vi "HandleObservation.vi"(8 "error in (no error)":errorcluster, 11 "S4ACS_GUI in":refnum<class "S4GUI.lvclass">) -> (0 "error out":errorcluster, 3 "S4ACS_GUI out":refnum<class "S4GUI.lvclass">)   [LabVIEW 2018, in "S4GUI.lvclass"]
uses:
  S4GUI.lvclass
  S4GUI.lvclass/S4GUI.ctl
  Acquisition/Acquisition.lvclass
  Trigger/Trigger.lvclass
  SyncBox/Sync Box.lvclass
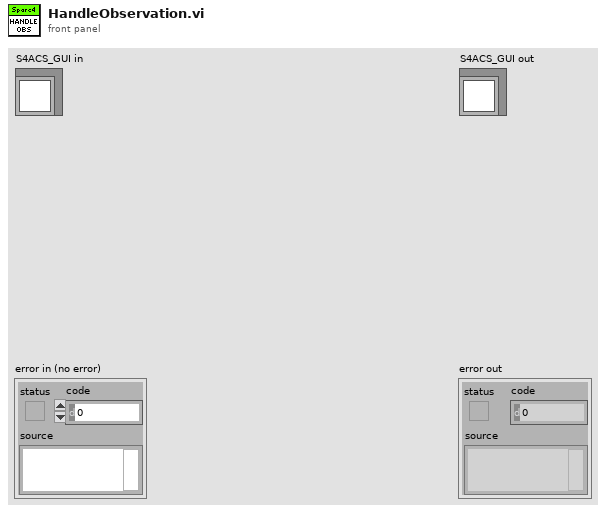
[diagram p1: front panel]
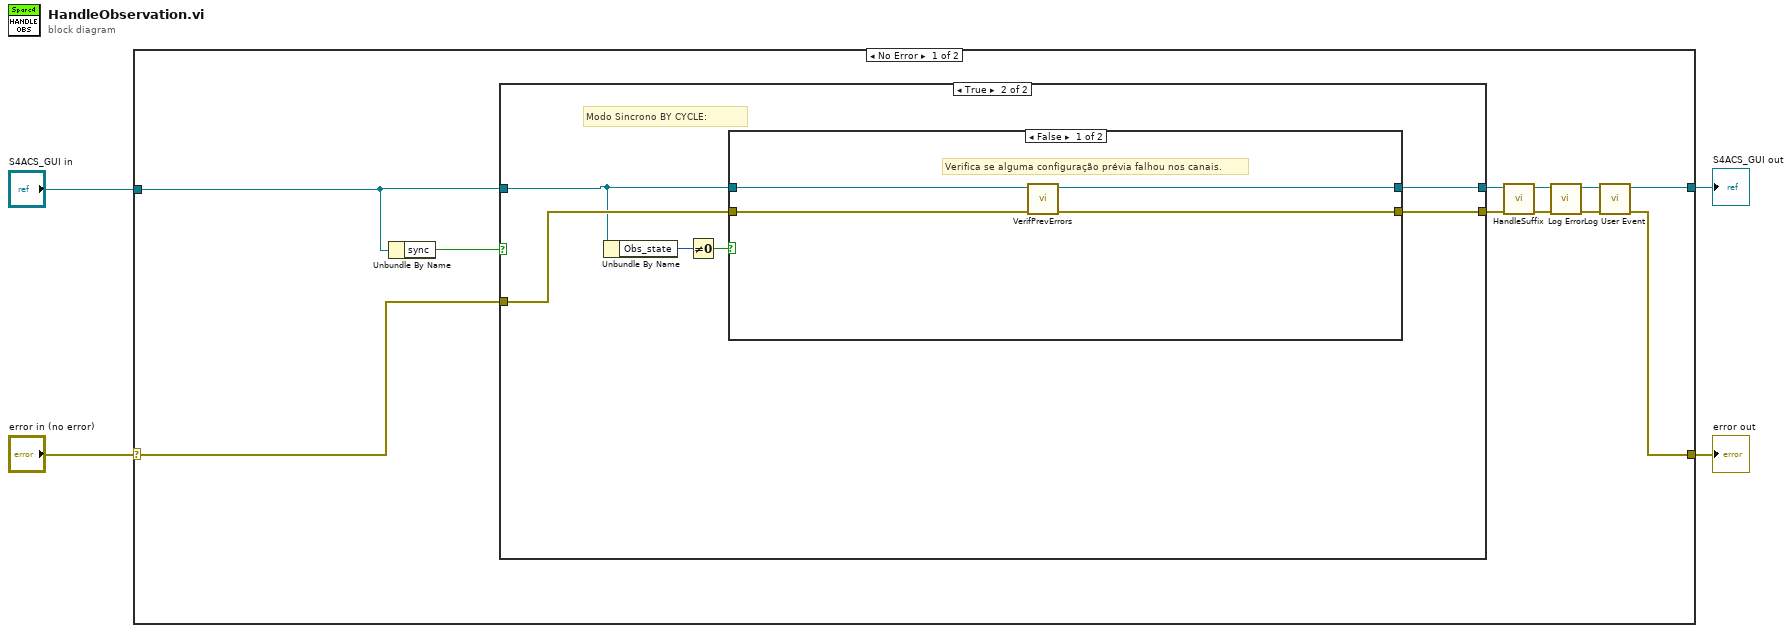
[diagram p0: block diagram]
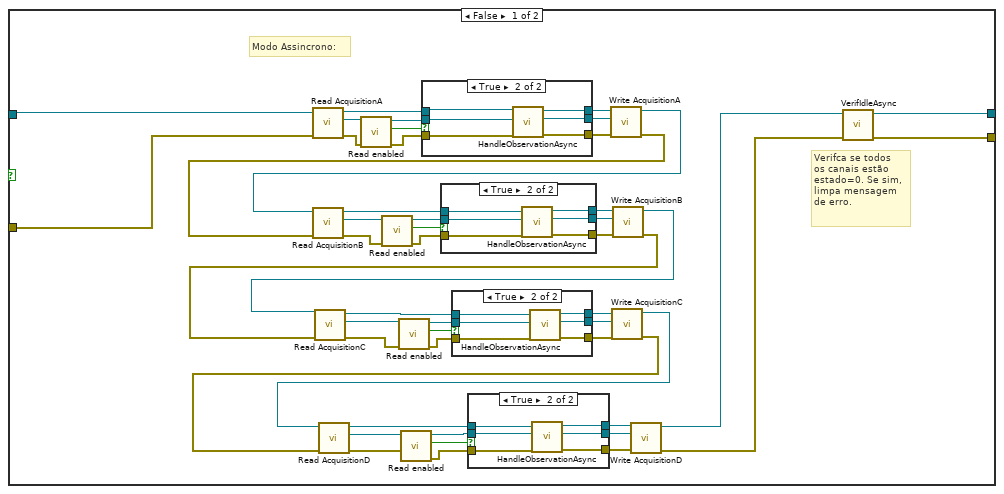
[diagram p2: hidden frame]
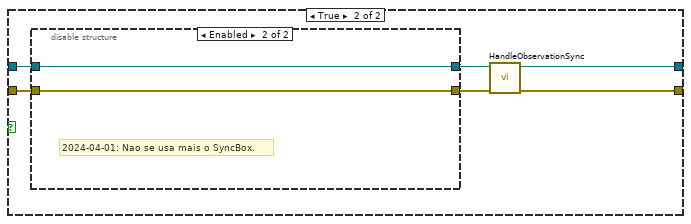
[diagram p7: hidden frame]
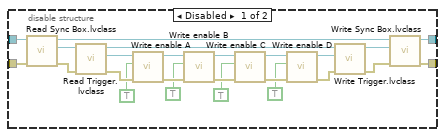
[diagram p8: hidden frame]
diagram:
  n1 = case shown="No Error" "error in (no error)" {
    selector: "error in (no error)" -> [w13 w143]
    tunnel: [w9 w143] -> w3
    tunnel: [w10 w142] -> w1
    tunnel: "S4ACS_GUI in" -> [w15 w142]
    frame No Error {
      n2 = Unbundle By Name(w15) -> ("sync"=w14:bool)
      n3 = case shown="True" w14 {
        tunnel: w15 -> [w27 w102]
        tunnel: [w17 w105] -> w8
        tunnel: w13 -> [w26 w103]
        tunnel: [w16 w104] -> w6
        frame False {
          # "Verifca se todos\nos canais estão \nestado=0. Se sim,\nlimpa mensagem \nde erro."
          # "Modo Assincrono:"
          n4 = call-dynamic "Read AcquisitionA.vi"("error in (no error)"=w26, "S4ACS_GUI in"=w27) -> ("error out"=w56:errorcluster, "Acquisition.lvclass"=w59:refnum<class "Acquisition.lvclass">, "S4ACS_GUI out"=w63:refnum<class "S4GUI.lvclass">)  [unwired: 7 in]
          n5 = call-dynamic "Read enabled.vi"("error in (no error)"=w56, "Server in"=w59) -> ("error out"=w55:errorcluster, "enabled"=w57:bool, "Server out"=w58:refnum<class "Acquisition.lvclass">)  [unwired: 7 in]
          n6 = case shown="True" w57 {
            tunnel: w63 -> [w92 w99]
            tunnel: w58 -> [w93 w98]
            tunnel: w55 -> [w91 w97]
            tunnel: [w92 w96] -> w62
            tunnel: [w93 w95] -> w61
            tunnel: [w91 w94] -> w60
            frame False {
            }
            frame True {
              n7 = call-dynamic "HandleObservationAsync.vi"("error in (no error)"=w97, "Acquisition.lvclass In"=w98, "S4ACS_GUI in"=w99) -> ("error out"=w94:errorcluster, "Acquisition.lvclass Out"=w95:refnum<class "Acquisition.lvclass">, "S4ACS_GUI out"=w96:refnum<class "S4GUI.lvclass">)  [unwired: 6 in]
            }
          }
          n8 = call-dynamic "Write AcquisitionA.vi"("error in (no error)"=w60, "Acquisition.lvclass"=w61, "S4ACS_GUI in"=w62) -> ("error out"=w24:errorcluster, "S4ACS_GUI out"=w25:refnum<class "S4GUI.lvclass">)  [unwired: 7 in]
          n9 = call "Read AcquisitionB.vi"("error in (no error)"=w24, "S4ACS_GUI in"=w25) -> ("error out"=w50:errorcluster, "Acquisition.lvclass"=w53:refnum<class "Acquisition.lvclass">, "S4ACS_GUI out"=w54:refnum<class "S4GUI.lvclass">)  [unwired: 7 in]
          n10 = call-dynamic "Read enabled.vi"("error in (no error)"=w50, "Server in"=w53) -> ("error out"=w49:errorcluster, "enabled"=w51:bool, "Server out"=w52:refnum<class "Acquisition.lvclass">)  [unwired: 7 in]
          n11 = case shown="True" w51 {
            tunnel: w54 -> [w83 w90]
            tunnel: w52 -> [w84 w89]
            tunnel: w49 -> [w82 w88]
            tunnel: [w83 w87] -> w46
            tunnel: [w84 w86] -> w47
            tunnel: [w82 w85] -> w48
            frame False {
            }
            frame True {
              n12 = call-dynamic "HandleObservationAsync.vi"("error in (no error)"=w88, "Acquisition.lvclass In"=w89, "S4ACS_GUI in"=w90) -> ("error out"=w85:errorcluster, "Acquisition.lvclass Out"=w86:refnum<class "Acquisition.lvclass">, "S4ACS_GUI out"=w87:refnum<class "S4GUI.lvclass">)  [unwired: 6 in]
            }
          }
          n13 = call "Write AcquisitionB.vi"("error in (no error)"=w48, "Acquisition.lvclass"=w47, "S4ACS_GUI in"=w46) -> ("error out"=w22:errorcluster, "S4ACS_GUI out"=w23:refnum<class "S4GUI.lvclass">)  [unwired: 7 in]
          n14 = call-dynamic "Read AcquisitionC.vi"("error in (no error)"=w22, "S4ACS_GUI in"=w23) -> ("error out"=w37:errorcluster, "Acquisition.lvclass"=w38:refnum<class "Acquisition.lvclass">, "S4ACS_GUI out"=w42:refnum<class "S4GUI.lvclass">)  [unwired: 7 in]
          n15 = call-dynamic "Read enabled.vi"("error in (no error)"=w37, "Server in"=w38) -> ("error out"=w43:errorcluster, "enabled"=w44:bool, "Server out"=w45:refnum<class "Acquisition.lvclass">)  [unwired: 7 in]
          n16 = case shown="True" w44 {
            tunnel: w42 -> [w74 w81]
            tunnel: w45 -> [w75 w80]
            tunnel: w43 -> [w73 w79]
            tunnel: [w74 w78] -> w41
            tunnel: [w75 w77] -> w40
            tunnel: [w73 w76] -> w39
            frame False {
            }
            frame True {
              n17 = call-dynamic "HandleObservationAsync.vi"("error in (no error)"=w79, "Acquisition.lvclass In"=w80, "S4ACS_GUI in"=w81) -> ("error out"=w76:errorcluster, "Acquisition.lvclass Out"=w77:refnum<class "Acquisition.lvclass">, "S4ACS_GUI out"=w78:refnum<class "S4GUI.lvclass">)  [unwired: 6 in]
            }
          }
          n18 = call-dynamic "Write AcquisitionC.vi"("error in (no error)"=w39, "Acquisition.lvclass"=w40, "S4ACS_GUI in"=w41) -> ("error out"=w20:errorcluster, "S4ACS_GUI out"=w21:refnum<class "S4GUI.lvclass">)  [unwired: 7 in]
          n19 = call-dynamic "Read AcquisitionD.vi"("error in (no error)"=w20, "S4ACS_GUI in"=w21) -> ("error out"=w32:errorcluster, "Acquisition.lvclass"=w31:refnum<class "Acquisition.lvclass">, "S4ACS_GUI out"=w33:refnum<class "S4GUI.lvclass">)  [unwired: 7 in]
          n20 = call-dynamic "Read enabled.vi"("error in (no error)"=w32, "Server in"=w31) -> ("error out"=w34:errorcluster, "enabled"=w35:bool, "Server out"=w36:refnum<class "Acquisition.lvclass">)  [unwired: 7 in]
          n21 = case shown="True" w35 {
            tunnel: w33 -> [w65 w72]
            tunnel: w36 -> [w66 w71]
            tunnel: w34 -> [w64 w70]
            tunnel: [w65 w69] -> w30
            tunnel: [w66 w68] -> w29
            tunnel: [w64 w67] -> w28
            frame False {
            }
            frame True {
              n22 = call-dynamic "HandleObservationAsync.vi"("error in (no error)"=w70, "Acquisition.lvclass In"=w71, "S4ACS_GUI in"=w72) -> ("error out"=w67:errorcluster, "Acquisition.lvclass Out"=w68:refnum<class "Acquisition.lvclass">, "S4ACS_GUI out"=w69:refnum<class "S4GUI.lvclass">)  [unwired: 6 in]
            }
          }
          n23 = call-dynamic "Write AcquisitionD.vi"("error in (no error)"=w28, "Acquisition.lvclass"=w29, "S4ACS_GUI in"=w30) -> ("error out"=w18:errorcluster, "S4ACS_GUI out"=w19:refnum<class "S4GUI.lvclass">)  [unwired: 7 in]
          n24 = call-dynamic "VerifIdleAsync.vi"("error in (no error)"=w18, "S4GUI in"=w19) -> ("error out"=w16:errorcluster, "S4GUI out"=w17:refnum<class "S4GUI.lvclass">)  [unwired: 8 in]
        }
        frame True {
          # "Modo Sincrono BY CYCLE:"
          n25 = Unbundle By Name(w102) -> ("Obs_state"=w101:u32)
          n26 = Not Equal To 0?(x=w101) -> (x != 0?=w100:bool)
          n27 = case shown="False" w100 {
            tunnel: [w107 w115] -> w105
            tunnel: [w106 w114] -> w104
            tunnel: w102 -> [w109 w113]
            tunnel: w103 -> [w108 w112]
            frame False {
              # "Verifica se alguma configuração prévia falhou nos canais."
              n28 = call-dynamic "VerifPrevErrors.vi"("error in (no error)"=w108, "S4GUI in"=w109) -> ("error out"=w106:errorcluster, "S4GUI out"=w107:refnum<class "S4GUI.lvclass">)  [unwired: 8 in]
            }
            frame True {
              n29 = disable-structure shown="Enabled" {
                disable-tunnel: w113 -> [w119 w141]
                disable-tunnel: w112 -> [w118 w140]
                disable-tunnel: [w117 w140] -> w111
                disable-tunnel: [w116 w141] -> w110
                frame Disabled {
                  n30 = call-dynamic "Read Sync Box.lvclass.vi"("error in (no error)"=w118, "SPARC4_AC in"=w119) -> ("error out"=w130:errorcluster, "Sync Box.lvclass"=w139:refnum<class "Sync Box.lvclass">, "SPARC4_AC out"=w131:refnum<class "S4GUI.lvclass">)  [unwired: 7 in]
                  n31 = call-dynamic "Read Trigger.lvclass.vi"("error in (no error)"=w130, "Sync Box in"=w139) -> ("error out"=w129:errorcluster, "Trigger.lvclass"=w138:refnum<class "Trigger.lvclass">, "Sync Box out"=w136:refnum<class "Sync Box.lvclass">)  [unwired: 7 in]
                  n32 = call "Write enable A.vi"("error in (no error)"=w129, "enable A"=TRUE, "Trigger in"=w138) -> ("error out"=w128:errorcluster, "Trigger out"=w137:refnum<class "Trigger.lvclass">)  [unwired: 7 in]
                  n33 = call "Write enable B.vi"("error in (no error)"=w128, "enable B"=TRUE, "Trigger in"=w137) -> ("error out"=w127:errorcluster, "Trigger out"=w135:refnum<class "Trigger.lvclass">)  [unwired: 7 in]
                  n34 = call "Write enable C.vi"("error in (no error)"=w127, "enable C"=TRUE, "Trigger in"=w135) -> ("error out"=w126:errorcluster, "Trigger out"=w134:refnum<class "Trigger.lvclass">)  [unwired: 7 in]
                  n35 = call "Write enable D.vi"("error in (no error)"=w126, "enable D"=TRUE, "Trigger in"=w134) -> ("error out"=w125:errorcluster, "Trigger out"=w133:refnum<class "Trigger.lvclass">)  [unwired: 7 in]
                  n36 = call-dynamic "Write Trigger.lvclass.vi"("error in (no error)"=w125, "Trigger.lvclass"=w133, "Sync Box in"=w136) -> ("error out"=w124:errorcluster, "Sync Box out"=w132:refnum<class "Sync Box.lvclass">)  [unwired: 7 in]
                  n37 = call-dynamic "Write Sync Box.lvclass.vi"("error in (no error)"=w124, "Sync Box.lvclass"=w132, "SPARC4_AC in"=w131) -> ("error out"=w117:errorcluster, "SPARC4_AC out"=w116:refnum<class "S4GUI.lvclass">)  [unwired: 7 in]
                }
                frame Enabled {
                  # "2024-04-01: Nao se usa mais o SyncBox."
                }
              }
              n38 = call-dynamic "HandleObservationSync.vi"("error in (no error)"=w111, "S4GUI in"=w110) -> ("error out"=w114:errorcluster, "S4GUI out"=w115:refnum<class "S4GUI.lvclass">)  [unwired: 8 in]
            }
          }
        }
      }
      n39 = call-dynamic "HandleSuffix.vi"("error in (no error)"=w6, "S4GUI in"=w8) -> ("error out"=w5:errorcluster, "S4GUI out"=w7:refnum<class "S4GUI.lvclass">)  [unwired: 8 in]
      n40 = call-dynamic "Log Error.vi"("error in (no error)"=w5, "S4GUI in"=w7) -> ("error out"=w11:errorcluster, "S4GUI out"=w12:refnum<class "S4GUI.lvclass">)  [unwired: 8 in]
      n41 = call-dynamic "Log User Event.vi"("error in (no error)"=w11, "S4GUI in"=w12) -> ("error out"=w9:errorcluster, "S4GUI out"=w10:refnum<class "S4GUI.lvclass">)  [unwired: 8 in]
    }
    frame Error {
    }
  }
  "error out" <- w3
  "S4ACS_GUI out" <- w1
